vi "SLM - Update Spots.vi"(8 "error in (no error)":errorcluster, 11 "Spots Cluster":T1 {"Spots Settings Array"."Phase" step=0.7753; "Spots Settings Array"."Intensity" step=0.1 format="%.3g"; "Spots Settings Array"."z" step=1e-06 format="%.2g"; "Spots Settings Array"."y" step=1e-06 format="%.3g"; "Spots Settings Array"."x" step=1e-06 format="%.3g"}) -> (0 "error out":errorcluster, 3 "Spots Cluster out":T1 {"Spots Settings Array"."Phase" step=0.7753; "Spots Settings Array"."Intensity" step=0.1 format="%.3g"; "Spots Settings Array"."z" step=1e-06 format="%.2g"; "Spots Settings Array"."y" step=1e-06 format="%.3g"; "Spots Settings Array"."x" step=1e-06 format="%.3g"}, 5 "finished":bool=TRUE)   [LabVIEW 2020]
uses:
  <userlib>/SLM/SLM Spots.ctl
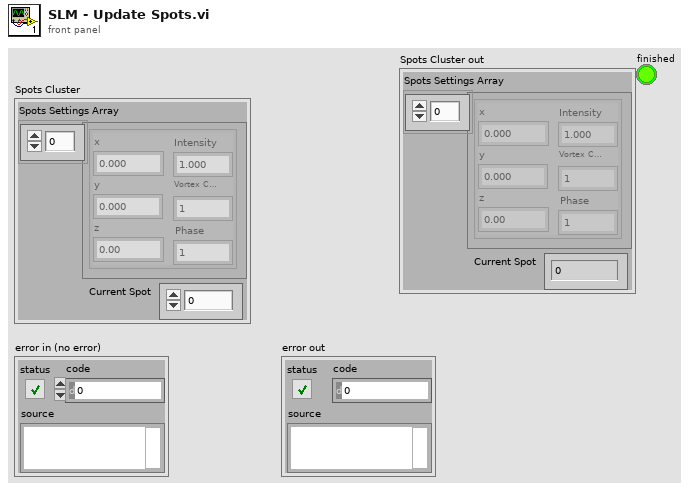
[diagram p1: front panel]
types:
  T1 = typedef "SLM Spots.ctl" = cluster{"Spots Settings Array":cluster{"x":dbl, "y":dbl, "z":dbl, "Intensity":dbl, "Vortex Charge":i8, "Phase":dbl}[], "Current Spot":i32}
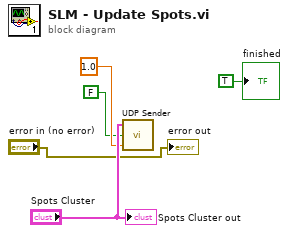
[diagram p0: block diagram]
diagram:
  n1 = call "UDP Sender.vi"("boost"=1.0, "Show panel"=FALSE, "Spots"="Spots Cluster") -> ()  [unwired: 1 out]
  "error out" <- "error in (no error)"
  "Spots Cluster out" <- "Spots Cluster"
  "finished" <- TRUE
